vi "Find and Rename VIs.vi"(8 "error in (no error)":errorcluster, 10 "New TLB Name":string, 11 "Owned Items[]":refnum<vi>[](array[refnum])) -> (0 "error out":errorcluster, 2 "Array 2":string[](array[string]), 3 "Array":string[](array[string]))   [LabVIEW 2015, in "TLB` Springboard.lvlib"]
uses:
  TLB` Springboard.lvlib
  <vilib>/regexp/Match Regular Expression.xnode
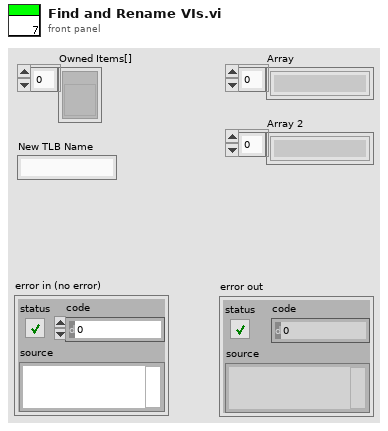
[diagram p1: front panel]
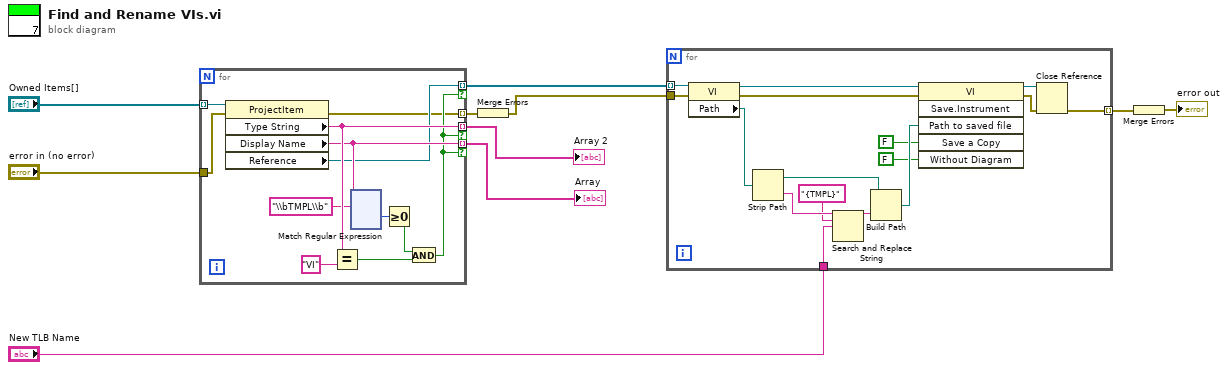
[diagram p0: block diagram]
diagram:
  n1 = for {
    tunnel: "Owned Items[]" -> [w22] mode=indexing
    tunnel: [w21] -> w4 mode=indexing if=w14
    tunnel: [w18] -> w5 mode=indexing if=w14
    tunnel: [w13] -> w8 mode=indexing if=w14
    tunnel: [w12] -> w9 mode=indexing
    tunnel: "error in (no error)" -> [w11]
    n2 = property class="ProjectItem"(reference=w22, error in=w11) -> (error out=w12:errorcluster, "Type String"=w21:string, "Display Name"=w18:string, "Reference"=w13:refnum<vi>)  [unwired: 1 out]
    n3 = Equal?(x=w21, y="VI") -> (x = y?=w19:bool)
    n4 = xnode "Match Regular Expression"("input string"=w18, "regular expression"="\\bTMPL\\b") -> ("offset past match"=w16:i32)  [unwired: 4 in, 4 out]
    n5 = Greater Or Equal To 0?(x=w16) -> (x >= 0?=w15:bool)
    n6 = And(x=w15, y=w19) -> (x .and. y?=w14:bool)
  }
  "Array" <- w5
  "Array 2" <- w4
  n7 = Merge Errors(w9) -> (w10:errorcluster)
  n8 = for {
    tunnel: "New TLB Name" -> [w149]
    tunnel: w8 -> [w144] mode=indexing
    tunnel: w10 -> [w138]
    tunnel: [w137] -> w2 mode=indexing
    n9 = property class="VI"(reference=w144, error in=w138) -> (reference out=w152:refnum<vi>, error out=w139:errorcluster, "Path"=w151:path)
    n10 = Strip Path(path=w151) -> (stripped path=w147:path, name=w150:string)
    n11 = Search and Replace String(input string=w150, search string="{TMPL}", replace string=w149) -> (result string=w146:string)  [unwired: 5 in, 3 out]
    n12 = Build Path(base path=w147, name or relative path=w146) -> (appended path=w145:path)
    n13 = invoke class="VI" method="Save.Instrument"(reference=w152, error in=w139, "Path to saved file"=w145, "Save a Copy"=FALSE, "Without Diagram"=FALSE) -> (reference out=w141:refnum<vi>, error out=w140:errorcluster)  [unwired: 1 in, 4 out]
    n14 = Close Reference(reference=w141, error in (no error)=w140) -> (error out=w137:errorcluster)
  }
  n15 = Merge Errors(w2) -> (→"error out":errorcluster)
